vi "SparkFun_AccelerometerADXL345_I2C_Open.vi"(7 "I2C Bus":T2, 8 "error in":errorcluster, 9 "Accel Range":T1 items=["+/- 2 g", "+/- 4 g", "+/- 8 g", "+/- 16 g"], 10 "ADXL345 Axes":T3={"X-Axis"=TRUE, "Y-Axis"=FALSE, "Z-Axis"=FALSE}, 11 "Controller":T4) -> (0 "error out":errorcluster, 3 "AccelerometerDevRef":T5={"DevStatus"={"status"=FALSE, "code"=0, "source"=""}, "Controller"=enum."Controller 1", "Scaling"={"Gain (VoltsPerG)"=0.0, "Center Voltage"=0.0}, "Analog Channels"={"X-Axis"=enum."Invalid", "Y-Axis"=enum."Invalid", "Z-Axis"=enum."Invalid"}, "I2C Bus"=enum."Invalid", "SPI Bus"=enum."Invalid", "Accel Range"=0, "ADXL345 Axes"={"X-Axis"=FALSE, "Y-Axis"=FALSE, "Z-Axis"=FALSE}, "Handle"=0, "Device Address"=0, "Accel Type"=enum."Analog"} {"Device Address" format="%.0x"; "Accel Range" items=["+/- 2 g", "+/- 4 g", "+/- 8 g", "+/- 16 g"]})   [LabVIEW 2014]
doc: "Opens a reference to the accelerometer you specify. You must open a reference before using any other VIs on this palette.\n\nThis software is licensed. Open the labview\\readme\\WPI Robotics Library Open Source License.txt file for more information."
uses:
  <vilib>/Rock Robotics/WPI/Accelerometer/WPI_AccelerometerDevRef.ctl
  <vilib>/Rock Robotics/SystemInterfaces/Typedef/FPGA_TypedefAnalogModule.ctl
  <vilib>/Rock Robotics/WPI/Accelerometer/WPI_AccelerometerScaling.ctl
  <vilib>/Rock Robotics/WPI/Accelerometer/WPI_AccelerometerAnalogChannels.ctl
  <vilib>/Rock Robotics/SystemInterfaces/AI/FPGA_AIChannel.ctl
  <vilib>/Rock Robotics/SystemInterfaces/i2clib/i2c_bus.ctl
  <vilib>/Rock Robotics/SystemInterfaces/spilib/spi_bus.ctl
  <vilib>/Rock Robotics/WPI/Accelerometer/ADXL345 Range.ctl
  <vilib>/Rock Robotics/WPI/Accelerometer/WPI_AccelerometerADXL345 Axes.ctl
  <vilib>/Rock Robotics/SystemInterfaces/NetworkCommunication/NetComm_UsageReport_ResourceType.ctl
panel:
  # "ADXL345"
  # "Analog"
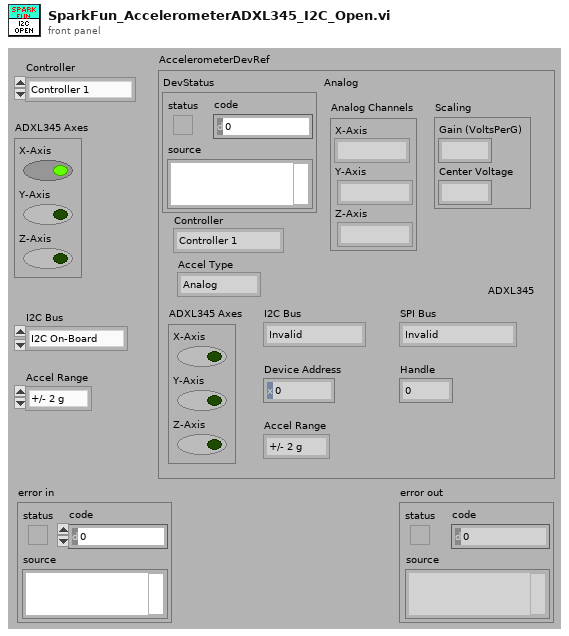
[diagram p1: front panel]
types:
  T1 = typedef "ADXL345 Range.ctl" = u8
  T2 = typedef "i2c_bus.ctl" = enum16{"I2C On-Board", "I2C MXP", "Invalid"}
  T3 = typedef "WPI_AccelerometerADXL345 Axes.ctl" = cluster{"X-Axis":bool, "Y-Axis":bool, "Z-Axis":bool}
  T4 = typedef "FPGA_TypedefAnalogModule.ctl" = enum16{"Controller 1"}
  T5 = typedef "WPI_AccelerometerDevRef.ctl" = cluster{"DevStatus":errorcluster, "Controller":T4, "Scaling":T6, "Analog Channels":T7, "I2C Bus":T2, "SPI Bus":T9, "Accel Range":T1, "ADXL345 Axes":T3, "Handle":i32, "Device Address":u8, "Accel Type":enum16{"Analog", "ADXL345 I2C", "ADXL345 SPI", "Internal"}}
  T6 = typedef "WPI_AccelerometerScaling.ctl" = cluster{"Gain (VoltsPerG)":dbl, "Center Voltage":dbl}
  T7 = typedef "WPI_AccelerometerAnalogChannels.ctl" = cluster{"X-Axis":T8, "Y-Axis":T8, "Z-Axis":T8}
  T8 = typedef "FPGA_AIChannel.ctl" = enum8{"AI 0", "AI 1", "AI 2", "AI 3", "AI MXP 0", "AI MXP 1", "AI MXP 2", "AI MXP 3", "Invalid"}
  T9 = typedef "spi_bus.ctl" = enum16{"SPI On-Board, CS0", "SPI On-Board, CS1", "SPI On-Board, CS2", "SPI On-Board, CS3", "SPI MXP", "Invalid"}
  T10 = typedef "NetComm_UsageReport_ResourceType.ctl" = enum8{"Controller", "Module", "Language", "CANPlugin", "Accelerometer", "ADXL345", "AnalogChannel", "AnalogTrigger", "AnalogTriggerOutput", "CANJaguar", "Compressor", "Counter", "Dashboard", "DigitalInput", "DigitalOutput", "DriverStationCIO", "DriverStationEIO", "DriverStationLCD", "Encoder", "GearTooth", "Gyro", "I2C", "Framework", "Jaguar", "Joystick", "Kinect", "KinectStick", "PIDController", "Preferences", "PWM", "Relay", "RobotDrive", "SerialPort", "Servo", "Solenoid", "SPI", "Task", "Ultrasonic", "Victor", "Button", "Command", "AxisCamera", "PCVideoServer", "SmartDashboard", "Talon", "HiTechnicColorSensor", "HiTechnicAccel", "HiTechnicCompass", "SRF08", "AnalogOutput", "Victor SP", "Talon SRX", "CAN Talon SRX"}
  T11 = typedef "WPI_I2CDevRef.ctl" = cluster{"DevStatus":errorcluster, "Controller":T12, "Device Address":u8, "Handle":i32, "I2C Bus":T2}
  T12 = typedef "FPGA_TypedefDigitalModule.ctl" = enum16{"Controller 1"}
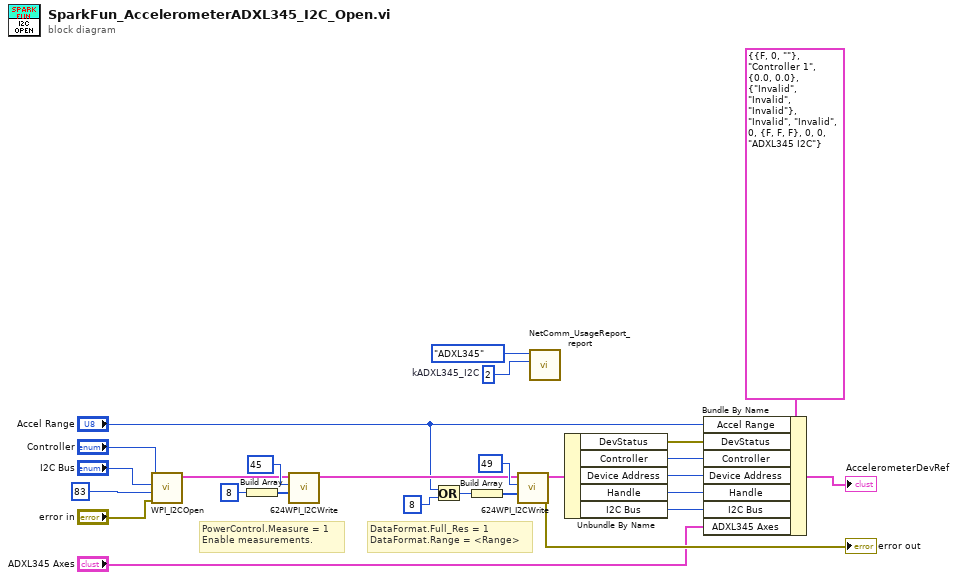
[diagram p0: block diagram]
diagram:
  w24 = u8 2  # kADXL345_I2C
  # "DataFormat.Full_Res = 1\nDataFormat.Range = <Range>"
  # "PowerControl.Measure = 1\nEnable measurements."
  n1 = call <vilib>:"WPI_I2COpen.vi"("error in"="error in", "Device Address"=u8 83, "I2C Bus"="I2C Bus", "Controller"="Controller") -> ("I2CDevRef"=w16:T11)  [unwired: 7 out]
  n2 = Build Array(u8 8 ("Data To Send")) -> (w19:u8[])
  n3 = call "624WPI_I2CWrite.vi"("I2CDataToSend"=w19, "I2CRegister"=u8 45 ("Data To Send"), "I2CDevRef"=w16) -> ("I2CDevRef"=w15:T11)  [unwired: 1 in, 7 out]
  n4 = Or(x="Accel Range", y=u8 8 ("Data To Send")) -> (x .or. y?=w20:T1)
  n5 = Build Array(w20) -> (w21:T1[])
  n6 = call "624WPI_I2CWrite.vi"("I2CDataToSend"=w21, "I2CRegister"=u8 49 ("Data To Send"), "I2CDevRef"=w15) -> ("error out"=→"error out":errorcluster, "I2CDevRef"=w11:T11)  [unwired: 1 in, 6 out]
  n7 = call <vilib>:"NetComm_UsageReport_report.vi"("Instance Number"=w24, "Resource Type"=NetComm_UsageReport_ResourceType."ADXL345") -> ()  [unwired: 10 in]
  n8 = Unbundle By Name(w11) -> ("DevStatus"=w9:errorcluster, "Controller"=w8:T12, "Device Address"=w3:u8, "Handle"=w6:i32, "I2C Bus"=w7:T2)
  n9 = Bundle By Name(cluster=T5 {"DevStatus"={"status"=FALSE, "code"=0, "source"=""}, "Controller"=enum."Controller 1", "Scaling"={"Gain (VoltsPerG)"=0.0, "Center Voltage"=0.0}, "Analog Channels"={"X-Axis"=enum."Invalid", "Y-Axis"=enum."Invalid", "Z-Axis"=enum."Invalid"}, "I2C Bus"=enum."Invalid", "SPI Bus"=enum."Invalid", "Accel Range"=0, "ADXL345 Axes"={"X-Axis"=FALSE, "Y-Axis"=FALSE, "Z-Axis"=FALSE}, "Handle"=0, "Device Address"=0, "Accel Type"=enum."ADXL345 I2C"} ("AccelerometerDevRef"), "Accel Range"="Accel Range", "DevStatus"=w9, "Controller"=w8, "Device Address"=w3, "Handle"=w6, "I2C Bus"=w7, "ADXL345 Axes"="ADXL345 Axes") -> (→"AccelerometerDevRef":T5)
